vi "Read Spawn Rate.vi"(8 "error in (no error)":errorcluster, 11 "Hungry Wolf in":refnum<class "Hungry Wolf.lvclass">) -> (0 "error out":errorcluster, 2 "Spawn Rate":dbl=0.03, 3 "Hungry Wolf out":refnum<class "Hungry Wolf.lvclass">)   [LabVIEW 2014, in "Hungry Wolf.lvclass"]
uses:
  Hungry Wolf.lvclass
  Hungry Wolf.lvclass/Hungry Wolf.ctl
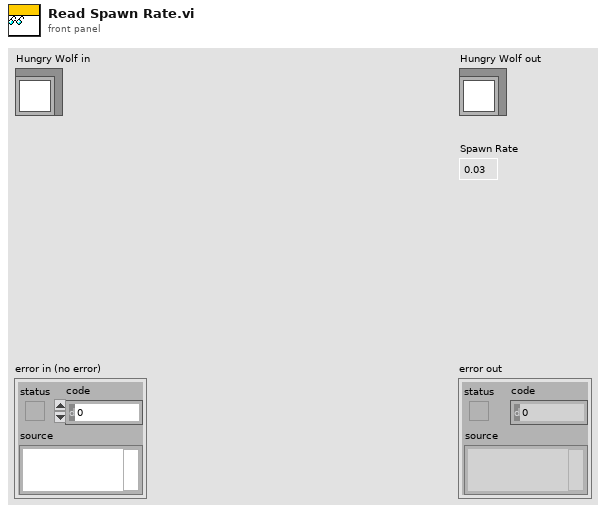
[diagram p1: front panel]
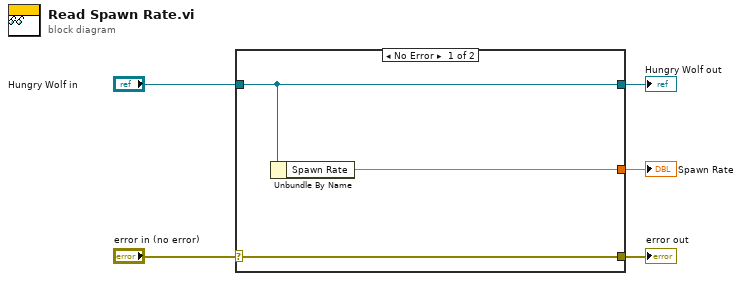
[diagram p0: block diagram]
diagram:
  n1 = case shown="No Error" "error in (no error)" {
    selector: "error in (no error)" -> [w8 w9]
    tunnel: [w8 w9] -> w4
    tunnel: [w7 w10] -> w2
    tunnel: "Hungry Wolf in" -> [w7 w10]
    tunnel: [w6 _] -> w1
    frame No Error {
      n2 = Unbundle By Name(w7) -> ("Spawn Rate"=w6:dbl)
    }
    frame Error {
    }
  }
  "error out" <- w4
  "Hungry Wolf out" <- w2
  "Spawn Rate" <- w1
